vi "determineBaseConfigPath.vi"(8 "error in (no error)":errorcluster, 11 "ConfigurationFileReader in":refnum<class "ConfigurationFileReader.lvclass">) -> (0 "error out":errorcluster, 2 "baseConfigPath":path, 3 "ConfigurationFileReader out":refnum<class "ConfigurationFileReader.lvclass">)   [LabVIEW 2016, in "Settings.lvlib" / "ConfigurationFileReader.lvclass"]
uses:
  ConfigurationFileReader.lvclass
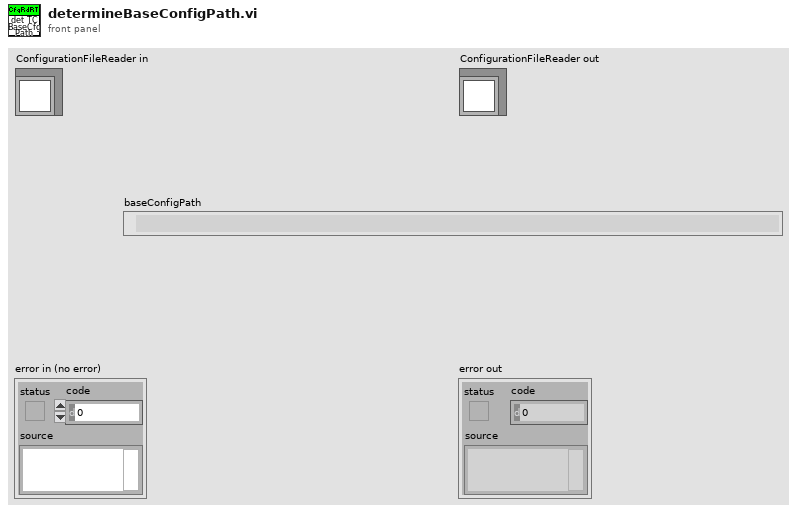
[diagram p1: front panel]
types:
  T1 = enum32{"invalid app kind", "Development System", "Run Time System", "Student Edition", "Embedded LabVIEW", "Evaluation", "Custom"}
  T2 = enum32{"invalid OS target", "Mac OS", "Windows 3.1", "Windows 95/NT", "Solaris 1", "Solaris 2", "HP-UX", "PowerMAX", "Linux", "Irix", "Rhapsody", "BeOS", "AIX", "OSF1", "VxWorks", "PharLap", "Carbon", "RTX", "Windows x64", "Linux x64", "Mac OS X x64"}
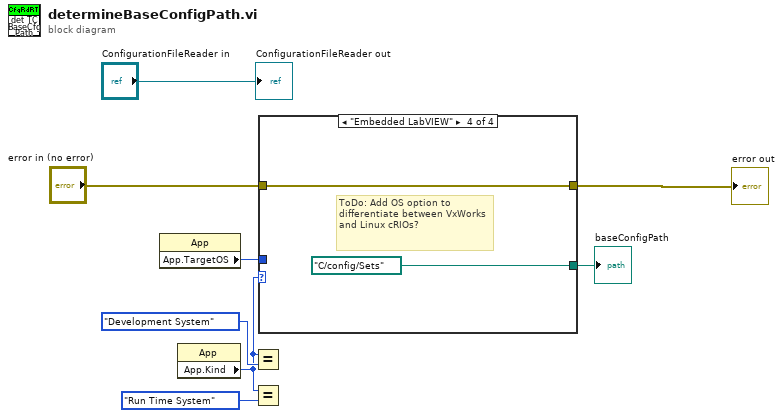
[diagram p0: block diagram]
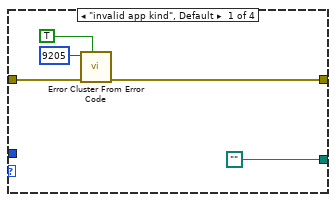
[diagram p2: hidden frame]
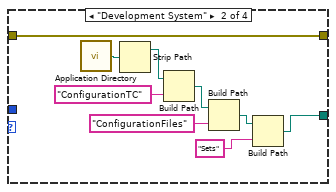
[diagram p3: hidden frame]
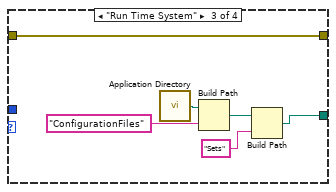
[diagram p4: hidden frame]
diagram:
  n1 = property class="App"() -> ("App.TargetOS"=w4:T2)  [unwired: 2 in, 2 out]
  n2 = property class="App"() -> ("App.Kind"=w5:T1)  [unwired: 2 in, 2 out]
  n3 = Equal?(x=w5, y=T1."Development System") -> ()  [unwired: 1 out]
  n4 = Equal?(x=w5, y=T1."Run Time System") -> ()  [unwired: 1 out]
  n5 = case shown="\"Embedded LabVIEW\"" w5 {
    tunnel: w4 -> [_ _ _ _]
    tunnel: [path "" w16 w24 path "C:/config/Sets" ("appended path")] -> w1
    tunnel: "error in (no error)" -> [w10 w17 w26 w29]
    tunnel: [w9 w17 w26 w29] -> w2
    frame "invalid app kind", Default {
      n6 = call <vilib>:"Error Cluster From Error Code.vi"("show call chain? (False)"=TRUE, "error in (no error)"=w10, "error code (0)"=9205) -> ("error out"=w9:errorcluster)  [unwired: 6 in]
    }
    frame "Development System" {
      n7 = call <vilib>:"Application Directory.vi"() -> ("Application Directory"=w20:path)
      n8 = Strip Path(path=w20) -> (stripped path=w22:path)  [unwired: 1 out]
      n9 = Build Path(base path=w22, name or relative path="ConfigurationTC") -> (appended path=w18:path)
      n10 = Build Path(base path=w18, name or relative path="ConfigurationFiles") -> (appended path=w15:path)
      n11 = Build Path(base path=w15, name or relative path="Sets") -> (appended path=w16:path)
    }
    frame "Run Time System" {
      n12 = call <vilib>:"Application Directory.vi"() -> ("Application Directory"=w27:path)
      n13 = Build Path(base path=w27, name or relative path="ConfigurationFiles") -> (appended path=w25:path)
      n14 = Build Path(base path=w25, name or relative path="Sets") -> (appended path=w24:path)
    }
    frame "Embedded LabVIEW" {
      # "ToDo: Add OS option to differentiate between VxWorks and Linux cRIOs?"
    }
  }
  "error out" <- w2
  "baseConfigPath" <- w1
  "ConfigurationFileReader out" <- "ConfigurationFileReader in"
